vi "GetLayersMaterialsFromSeparatedLayers.vi"(8 "error in (no error)":errorcluster, 10 "OutputFolder":path, 11 "Path_to_Tiff":path) -> (0 "error out":errorcluster, 1 "Layers":string[](array[string]), 2 "LayerNo":string[](array[string]), 3 "Materials":string[](array[string]), 4 "Separated Layer bmp []":path[](array[path]))   [LabVIEW 2022 SP3, in "TopLevel.lvclass"]
uses:
  TopLevel.lvclass
  <userlib>/_OpenG.lib/array/array.llb/Sort 1D Array (I32)__ogtk.vi
  <userlib>/_OpenG.lib/array/array.llb/Reorder 1D Array2 (Path)__ogtk.vi
  <userlib>/_OpenG.lib/array/array.llb/Reorder 1D Array2 (String)__ogtk.vi
panel:
  out "Sorted Array out":i32[](array[numeric])
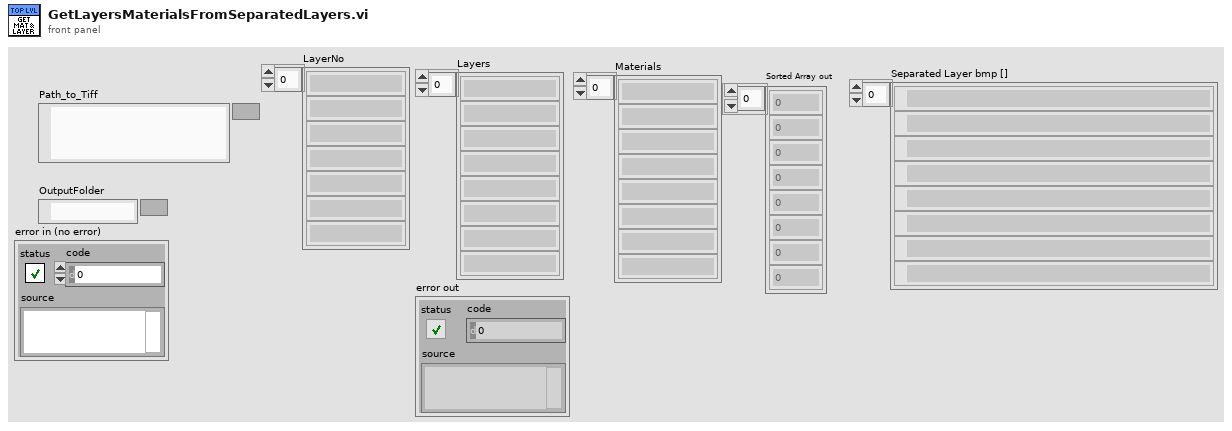
[diagram p1: front panel]
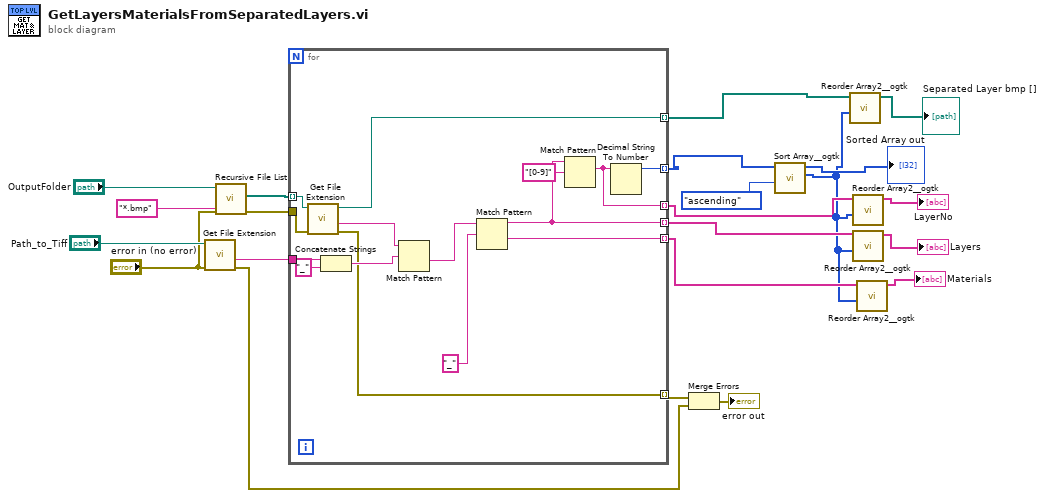
[diagram p0: block diagram]
diagram:
  n1 = call <vilib>:"Get File Extension.vi"("error in (no error)"="error in (no error)", "file"="Path_to_Tiff") -> ("error out"=w14:errorcluster, "filename without extension"=w22:string)  [unwired: 5 in, 3 out]
  n2 = call <vilib>:"Recursive File List.vi"("pattern"="*.bmp", "error in (no error)"="error in (no error)", "Folder Path"="OutputFolder") -> ("error out"=w16:errorcluster, "All Files in Dir"=w21:path[])  [unwired: 4 in, 3 out]
  n3 = for {
    tunnel: w21 -> [w37] mode=indexing
    tunnel: w22 -> [w36]
    tunnel: [w29] -> w9 mode=indexing
    tunnel: [w30] -> w8 mode=indexing
    tunnel: [w24] -> w12 mode=indexing
    tunnel: w16 -> [w27]
    tunnel: [w26] -> w15 mode=indexing
    tunnel: [w25] -> w10 mode=indexing
    tunnel: [w23] -> w5 mode=indexing
    n4 = call <vilib>:"Get File Extension.vi"("error in (no error)"=w27, "file"=w37) -> ("error out"=w26:errorcluster, "filename without extension"=w32:string, "dup file"=w25:path)  [unwired: 5 in, 2 out]
    n5 = Concatenate Strings(w36, "_" ("string")) -> (w33:string)
    n6 = Match Pattern(string=w32, regular expression=w33) -> (after substring=w31:string)  [unwired: 1 in, 3 out]
    n7 = Match Pattern(string=w31, regular expression="_") -> (before substring=w29:string, after substring=w30:string)  [unwired: 1 in, 2 out]
    n8 = Match Pattern(string=w29, regular expression="[0-9]") -> (match substring=w23:string)  [unwired: 1 in, 3 out]
    n9 = Decimal String To Number(string=w23) -> (number=w24:i32)  [unwired: 2 in, 1 out]
  }
  n10 = Merge Errors(w15, w14) -> (→"error out":errorcluster)
  n11 = call-poly <userlib>:"Sort Array__ogtk.vi"("Order"=enum16{"ascending", "descending"}."ascending", "Array in"=w12) -> ("Sorted Pointers"=w1:i32[], "Sorted Array out"=→"Sorted Array out":i32[])  [unwired: 8 in]
  n12 = call-poly <userlib>:"Reorder Array2__ogtk.vi"("indices"=w1, "array"=w10) -> ("reordered array"=→"Separated Layer bmp []":path[])  [unwired: 9 in]
  n13 = call-poly <userlib>:"Reorder Array2__ogtk.vi"("indices"=w1, "array"=w5) -> ("reordered array"=→"LayerNo":string[])  [unwired: 9 in]
  n14 = call-poly <userlib>:"Reorder Array2__ogtk.vi"("indices"=w1, "array"=w9) -> ("reordered array"=→"Layers":string[])  [unwired: 9 in]
  n15 = call-poly <userlib>:"Reorder Array2__ogtk.vi"("indices"=w1, "array"=w8) -> ("reordered array"=→"Materials":string[])  [unwired: 9 in]
